vi "Step Calculation.vi"() -> ()   [LabVIEW 2018]
panel:
  out "Total steps/rotation":dbl
  out "Error In step":dbl
  out "Actual step angle":dbl
  out "Actual # steps required":dbl
  out "Step size":dbl
  out "# of step possible to move":dbl
  in  "Step Angle":dbl
  in  "# microstep/step":dbl
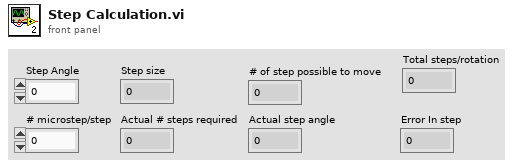
[diagram p1: front panel]
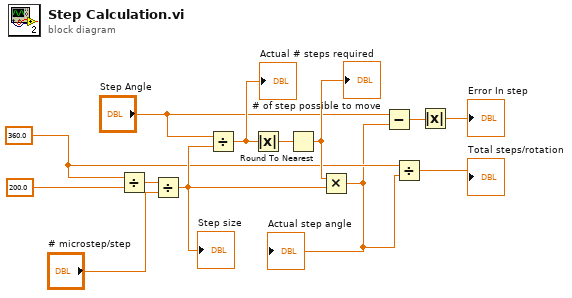
[diagram p0: block diagram]
diagram:
  w3 = 360.0 ("x")
  n1 = Divide(x=w3, y=200.0) -> (x/y=w12:dbl)
  n2 = Divide(x=w12, y="# microstep/step") -> (x/y=w10:dbl)
  "Step size" <- w10
  n3 = Divide(x="Step Angle", y=w10) -> (x/y=w8:dbl)
  "Actual # steps required" <- w8
  n4 = Absolute Value(x=w8) -> (abs(x)=w9:dbl)
  n5 = Round To Nearest(number=w9) -> (nearest integer value=w7:dbl)
  "# of step possible to move" <- w7
  n6 = Multiply(x=w7, y=w10) -> (x*y=w2:dbl)
  "Actual step angle" <- w2
  n7 = Subtract(x="Step Angle", y=w2) -> (x-y=w5:dbl)
  n8 = Divide(x=w3, y=w2) -> (x/y=→"Total steps/rotation":dbl)
  n9 = Absolute Value(x=w5) -> (abs(x)=→"Error In step":dbl)
